vi "system camera.vi"() -> ()   [LabVIEW 2016]
uses:
  <vilib>/userdefined/High Color/IMAQdx.ctl
  <vilib>/ErrorRing/Error Ring.xnode
  <vilib>/vision/driver/NI_Vision_Acquisition_Software.lvlib
panel:
  in  "input code given by the coustmer":string
  out "no treat":bool
  out "Image 2":T1(plugin-control)
  in  "File Path":path
  out "Image":T1(plugin-control)
  in  "Session In":T2
  in  "stop":bool
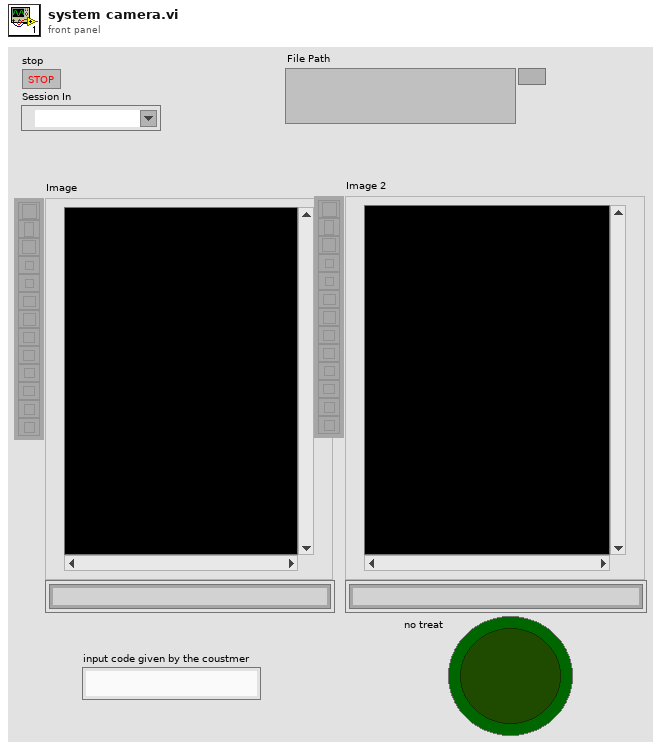
[diagram p1: front panel]
types:
  T1 = typedef "IMAQ Image.ctl" = refnum<image>
  T2 = typedef "IMAQdx.ctl" = refnum<k21>
  T3 = typedef "Image Type" = u32
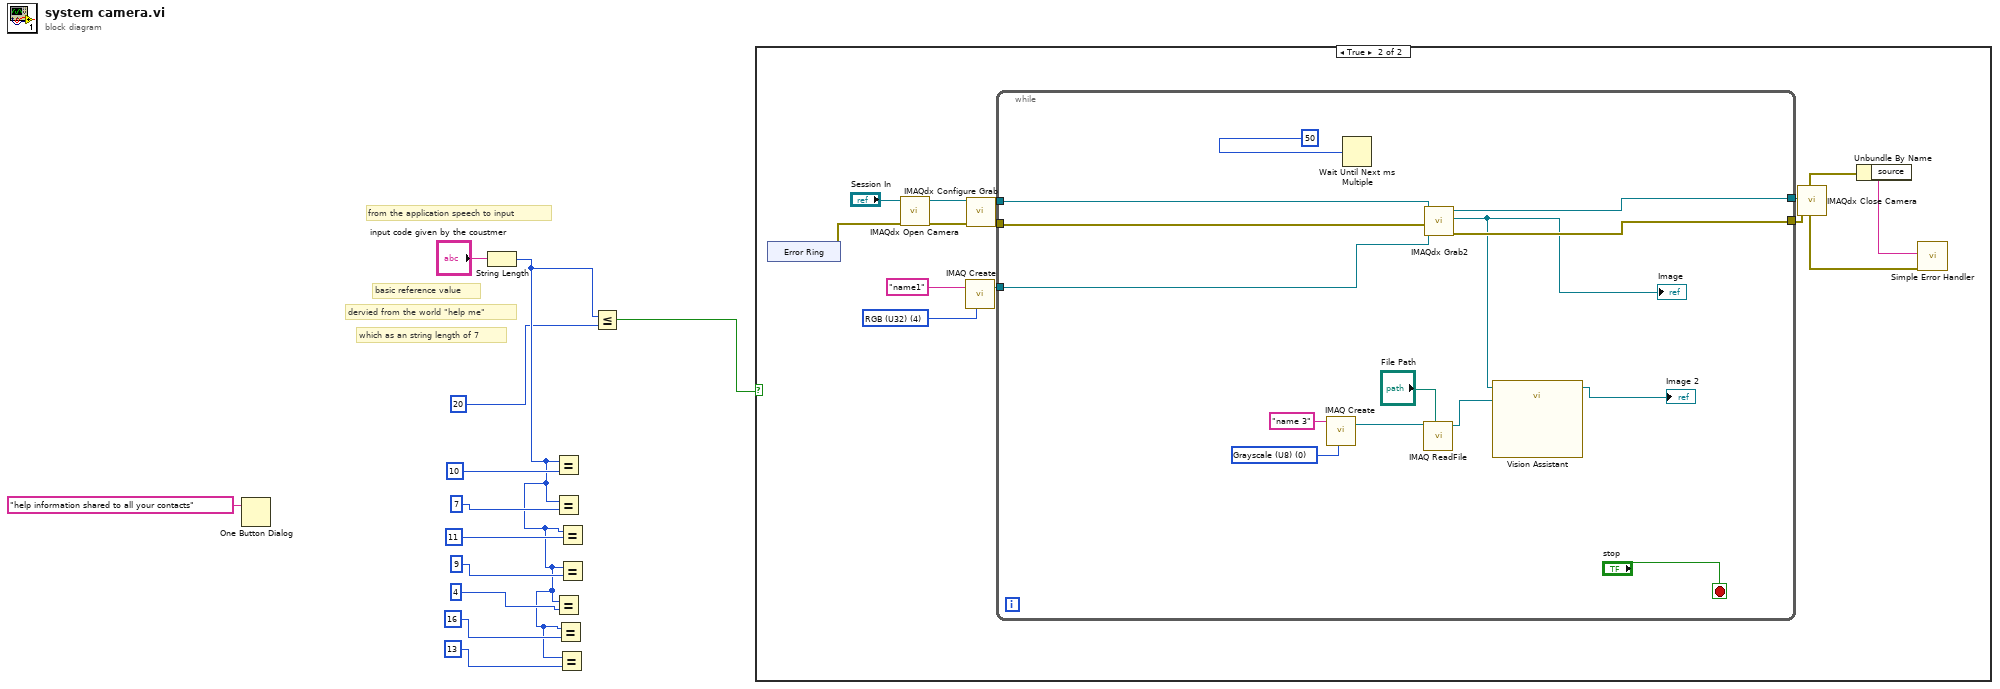
[diagram p0: block diagram]
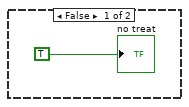
[diagram p2: hidden frame]
diagram:
  # "from the application speech to input"
  # "which as an string length of 7"
  # "dervied from the world \"help me\""
  # "basic reference value"
  n1 = One Button Dialog(message="help information shared to all your contacts") -> ()  [unwired: 1 in, 1 out]
  n2 = String Length(string="input code given by the coustmer") -> (length=w4:i32)
  n3 = Equal?(x=w4, y=10) -> ()  [unwired: 1 out]
  n4 = Equal?(x=w4, y=7) -> ()  [unwired: 1 out]
  n5 = Equal?(x=w4, y=4) -> ()  [unwired: 1 out]
  n6 = Equal?(x=w4, y=16) -> ()  [unwired: 1 out]
  n7 = Equal?(x=w4, y=13) -> ()  [unwired: 1 out]
  n8 = Equal?(x=w4, y=11) -> ()  [unwired: 1 out]
  n9 = Equal?(x=w4, y=9) -> ()  [unwired: 1 out]
  n10 = Less Or Equal?(x=w4, y=20) -> (x <= y?=w2:bool)
  n11 = case shown="True" w2 {
    frame False {
      "no treat" <- TRUE
    }
    frame True {
      w25 = T3 4 items=["Grayscale (U8)", "Grayscale (I16)", "Grayscale (SGL)", "Complex (CSG)", "RGB (U32)", "HSL (U32)", "RGB (U64)", "Grayscale (U16)"] ("Image Type")
      n12 = xnode "Error Ring"() -> ("error out"=w23:errorcluster)
      n13 = call <vilib>:"IMAQdx Open Camera.vi"("error in"=w23, "Session In"="Session In") -> ("error out"=w22:errorcluster, "Session Out"=w21:T2)  [unwired: 8 in]
      n14 = call "IMAQ Create"("Image Name"="name1", "Image Type"=w25) -> ("New Image"=w16:T1)  [unwired: 3 in, 1 out]
      n15 = call <vilib>:"IMAQdx Configure Grab.vi"("error in"=w22, "Session In"=w21) -> ("error out"=w19:errorcluster, "Session Out"=w20:T2)  [unwired: 8 in]
      n16 = while {
        tunnel: w20 -> [w41]
        tunnel: w19 -> [w40]
        tunnel: [w39] -> w18
        tunnel: [w38] -> w17
        tunnel: w16 -> [w37]
        stop <- "stop" stop-if-true
        w34 = T3 0 items=["Grayscale (U8)", "Grayscale (I16)", "Grayscale (SGL)", "Complex (CSG)", "RGB (U32)", "HSL (U32)", "RGB (U64)", "Grayscale (U16)"] ("Image Type")
        n17 = call "IMAQ Create"("Image Name"="name 3", "Image Type"=w34) -> ("New Image"=w33:T1)  [unwired: 3 in, 1 out]
        n18 = Wait Until Next ms Multiple(millisecond multiple=u32 50) -> ()  [unwired: 1 out]
        n19 = call "IMAQ ReadFile"("File Path"="File Path", "Image"=w33) -> ("Image Out"=w31:T1)  [unwired: 5 in, 4 out]
        n20 = call <vilib>:"IMAQdx Grab2.vi"("error in"=w40, "Image In"=w37, "Session In"=w41) -> ("error out"=w38:errorcluster, "Image Out"=w29:T1, "Session Out"=w39:T2)  [unwired: 5 in, 1 out]
        "Image" <- w29
        n21 = call "Vision Assistant"("Image In"=w29, "Image Dst"=w31) -> ("Image Out"=→"Image 2":T1)  [unwired: 23 in, 2 out]
      }
      n22 = call <vilib>:"IMAQdx Close Camera.vi"("error in"=w17, "Session In"=w18) -> ("error out"=w15:errorcluster)  [unwired: 9 in]
      n23 = Unbundle By Name(w15) -> ("source"=w14:string)
      n24 = call <vilib>:"Simple Error Handler.vi"("error source (\" \")"=w14, "error in (no error)"=w15) -> ()  [unwired: 3 in, 5 out]
    }
  }
